vi "List State Possible Owners.vi"(6 "Config Path(\"\" for lvcsm file)":path, 8 "error in (no error)":errorcluster, 11 "CSM States":string) -> (0 "Error out":errorcluster, 3 "possible owners":string[](array[string]))   [LabVIEW 2017, in "CSM-Helper API with lvcsm Support.lvlib"]
uses:
  CSM-Helper API with lvcsm Support.lvlib
  lvcsmFile/lvcsm File Path.vi
  <vilib>/Utility/config.llb/Open Config Data.vi
  <vilib>/Utility/config.llb/Get Section Names.vi
  <vilib>/Utility/config.llb/Close Config Data.vi
  lvcsmFile/lvcsm File Support.lvlib
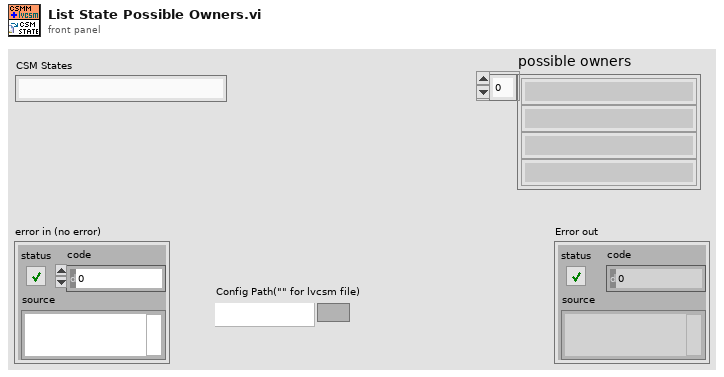
[diagram p1: front panel]
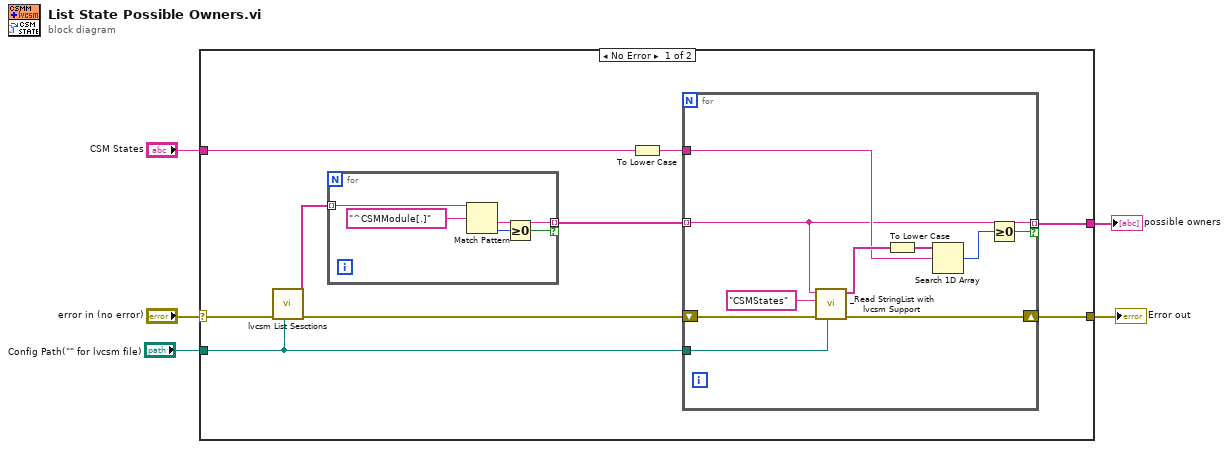
[diagram p0: block diagram]
diagram:
  n1 = case shown="No Error" "error in (no error)" {
    selector: "error in (no error)" -> [w14 w30]
    tunnel: [w10 w30] -> w5
    tunnel: "CSM States" -> [w9 _]
    tunnel: "Config Path(\"\" for lvcsm file)" -> [w7 _]
    tunnel: [w6 _] -> w1
    frame No Error {
      n2 = call "lvcsm List Sesctions.vi"("Config Path"=w7, "Error in"=w14) -> ("Error out"=w11:errorcluster, "section names"=w13:string[])  [unwired: 8 in]
      n3 = for {
        tunnel: w13 -> [w29] mode=indexing
        tunnel: [w27] -> w12 mode=indexing if=w26
        n4 = Match Pattern(string=w29, regular expression="^CSMModule[.]" ("Section")) -> (after substring=w27:string, offset past match=w25:i32)  [unwired: 1 in, 2 out]
        n5 = Greater Or Equal To 0?(x=w25) -> (x >= 0?=w26:bool)
      }
      n6 = To Lower Case(string=w9) -> (all lower case string=w8:string)
      n7 = for {
        tunnel: w12 -> [w16] mode=indexing
        shift-right: [w23] -> w10
        shift-left: w11 -> [w24]
        tunnel: [w16] -> w6 mode=indexing if=w20
        tunnel: w8 -> [w17]
        tunnel: w7 -> [w18]
        n8 = call "_Read StringList with lvcsm Support.vi"("Config Path(\"\" for lvcsm file)"=w18, "error in (no error)"=w24, "API Name"="CSMStates", "CSM Name"=w16) -> ("Error out"=w23:errorcluster, "CSMAPI List"=w22:string[])  [unwired: 6 in]
        n9 = To Lower Case(string=w22) -> (all lower case string=w21:string[])
        n10 = Search 1D Array(1D array=w21, element=w17) -> (index of element=w19:i32)  [unwired: 1 in]
        n11 = Greater Or Equal To 0?(x=w19) -> (x >= 0?=w20:bool)
      }
    }
    frame Error {
    }
  }
  "Error out" <- w5
  "possible owners" <- w1
